vi "Summation.vi"(7 "Reset":bool, 8 "Zone":i32, 11 "Number":dbl) -> (3 "sum":dbl)   [LabVIEW 2016]
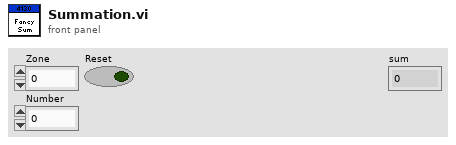
[diagram p1: front panel]
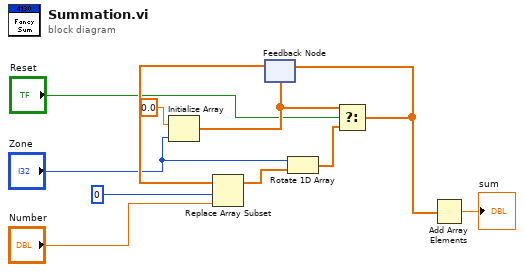
[diagram p0: block diagram]
diagram:
  n1 = Initialize Array(0.0 ("element"), "Zone") -> (w2:dbl[])
  n2 = feedback #1(w2) -> (w11:dbl[])
  n3 = Replace Array Subset(array=w11, new element="Number", index=0) -> (w10:dbl[])
  n4 = Rotate 1D Array(1:w10, 2:"Zone") -> (0:w3:dbl[])
  n5 = Select(t=w2, s="Reset", f=w3) -> (s? t:f=w4:dbl[])
  n6 = feedback-in #1(w4) -> ()
  n7 = Add Array Elements(numeric array=w4) -> (sum=→"sum":dbl)
